vi "Arcade Drive.vi"(4 "b":dbl=1.0, 5 "a":dbl=1.0, 7 "Metrics In":T1) -> (3 "Metrics Out":T1)   [LabVIEW 2015]
uses:
  Drive Train/Drive Metrics.ctl
  Drive Train/Drive States.ctl
  Drive Train/Copilot States.ctl
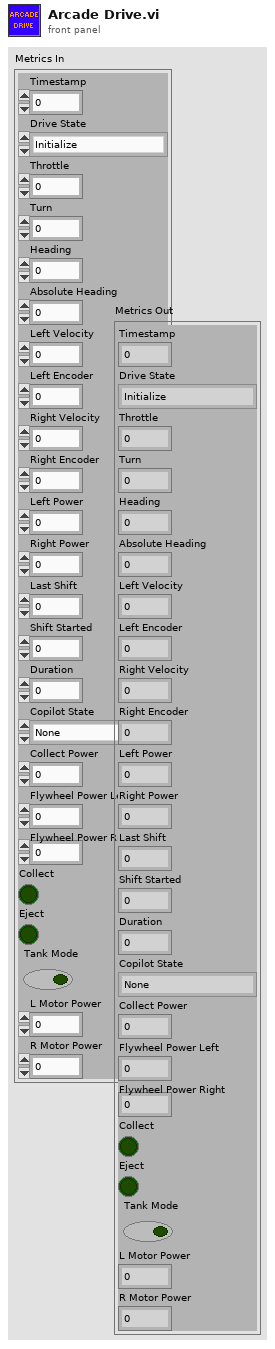
[diagram p1: front panel]
types:
  T1 = typedef "Drive Metrics.ctl" = cluster{"Timestamp":u32, "Drive State":T2, "Throttle":dbl, "Turn":dbl, "Heading":dbl, "Absolute Heading":dbl, "Left Velocity":dbl, "Left Encoder":dbl, "Right Velocity":dbl, "Right Encoder":dbl, "Left Power":dbl, "Right Power":dbl, "Last Shift":u32, "Shift Started":u32, "Duration":i64, "Copilot State":T3, "Collect Power":dbl, "Flywheel Power Left":dbl, "Flywheel Power Right":dbl, "Collect":bool, "Eject":bool, "Tank Mode":bool, "L Motor Power":dbl, "R Motor Power":dbl}
  T2 = typedef "Drive States.ctl" = enum16{"Initialize", "Low Gear", "Up Shift Begin", "Up Shifting", "Up Shift Delay", "High Gear", "Down Shift Begin", "Down Shifting", "Down Shift Delay"}
  T3 = typedef "Copilot States.ctl" = enum16{"None", "Lift collector", "Boulder to shooter", "Lifting collector", "Lifted Collector", "collected", "Collecting", "Ejecting", "dropping arm", "boulder ready", "shooter to angle", "flywheel spin up", "drop arm"}
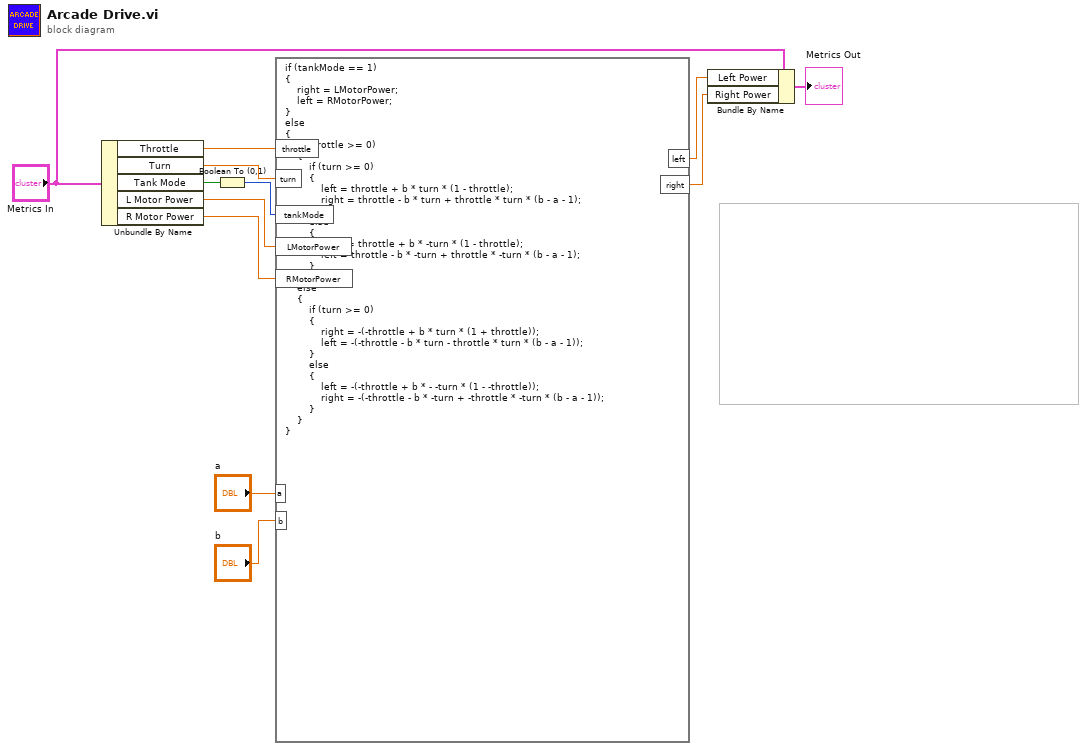
[diagram p0: block diagram]
diagram:
  n1 = Unbundle By Name("Metrics In") -> ("Throttle"=w10:dbl, "Turn"=w9:dbl, "Tank Mode"=w4:bool, "L Motor Power"=w2:dbl, "R Motor Power"=w1:dbl)
  n2 = Boolean To (0,1)(Boolean=w4) -> (0, 1=w3:i16)
  n3 = formula code="if (tankMode == 1)\n{\n    right = LMotorPower;\n    left = RMotorPower;\n} \nelse \n{\n   if (throttle >= 0)\n    {\n        if (turn >= 0)\n        {\n            left = throttle + b * turn * (1 - throttle);\n            right = throttle - b * turn + throttle * turn * (b - a - 1);\n        }\n        else\n        {\n            right = throttle + b * -turn * (1 - throttle);\n            left = throttle - b * -turn + throttle * -turn * (b - a - 1);\n        }\n    }\n    else\n    {\n        if (turn >= 0)\n        {\n            right = -(-throttle + b * turn * (1 + throttle));\n            left = -(-throttle - b * turn - throttle * turn * (b - a - 1));\n        }\n        else\n        {\n            left = -(-throttle + b * - -turn * (1 - -throttle));\n            right = -(-throttle - b * -turn + -throttle * -turn * (b - a - 1));\n        }\n    }\n}"("throttle"=w10, "turn"=w9, "a"="a", "b"="b", "tankMode"=w3, "LMotorPower"=w2, "RMotorPower"=w1) -> ("left"=w6:dbl, "right"=w5:dbl)
  n4 = Bundle By Name(cluster="Metrics In", "Left Power"=w6, "Right Power"=w5) -> (→"Metrics Out":T1)
